vi "Copy .LLB to NI VeriStand dir.vi"(5 "Files Generated by Build":path[](array[path]), 6 "Top Level/Always Included VIs":path[](array[path]), 7 "Destination Path":path, 8 "error in (no error)":errorcluster, 9 "Target Name":string, 10 "Build Specification Name":string, 11 "Project Path":path) -> (0 "error out":errorcluster)   [LabVIEW 2024]
doc: "This VI is called after each run of a build specification. The VI will copy the generated LLB (Engine or System Explorer) into the VeriStand Custom Device folder (...\\Documents\\National Instruments\\NI VeriStand 2013...)."
uses:
  NationalInstruments.VeriStand
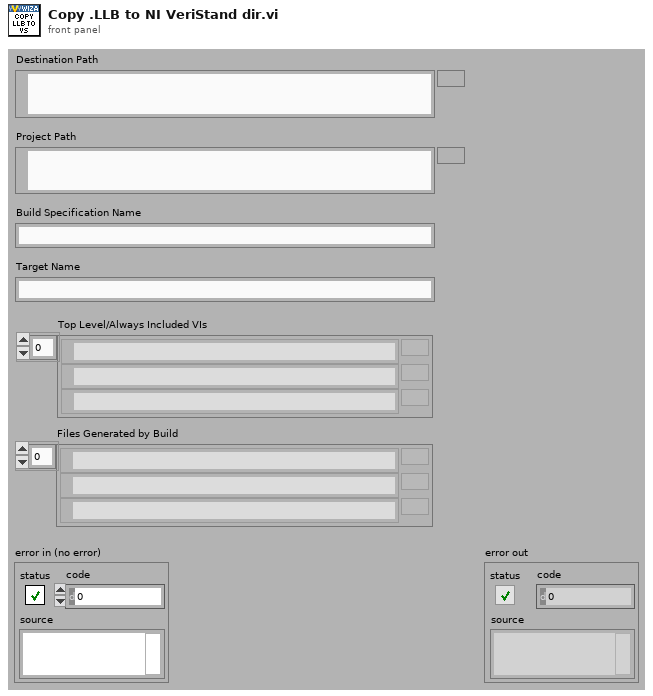
[diagram p1: front panel]
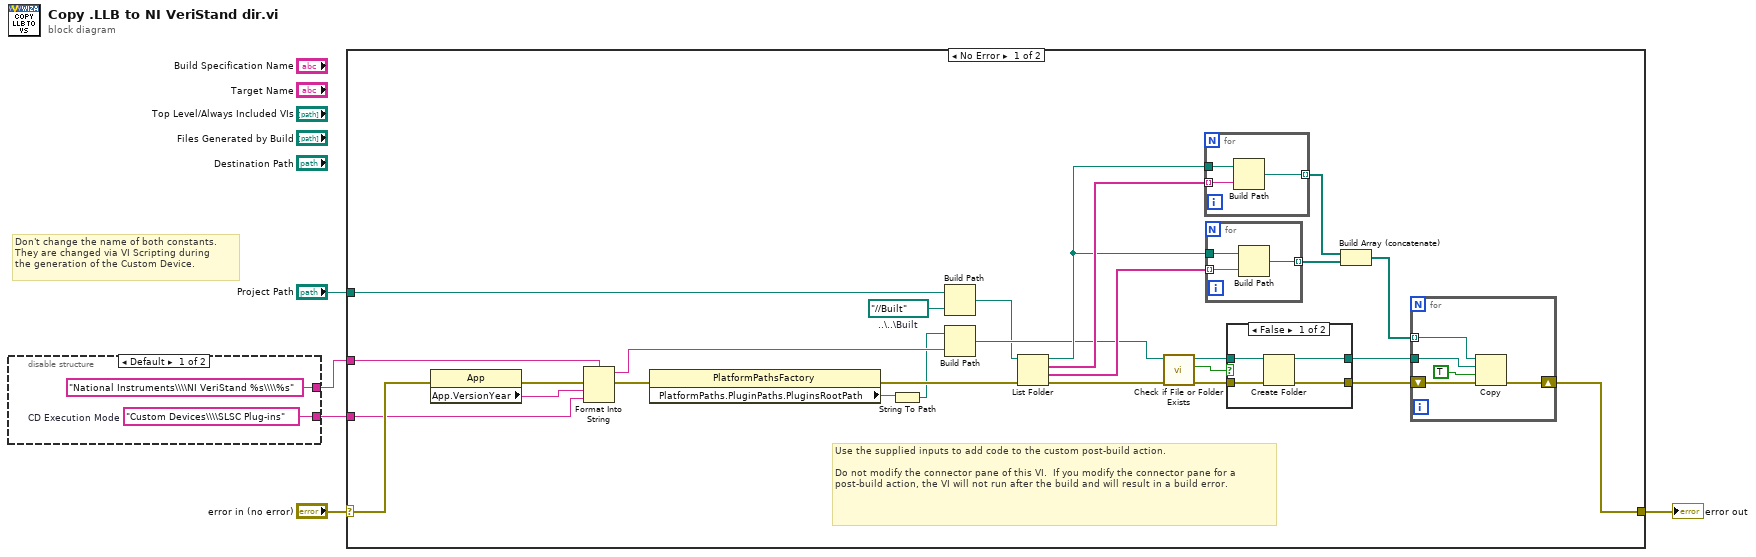
[diagram p0: block diagram]
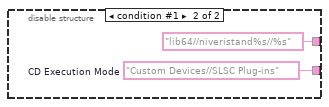
[diagram p4: hidden frame]
diagram:
  # "Don't change the name of both constants.\nThey are changed via VI Scripting during\nthe generation of the Custom Device."
  n1 = disable-structure shown="Default" {
    disable-tunnel: [w7 w9] -> w2
    disable-tunnel: ["National Instruments\\\\NI VeriStand %s\\\\%s" ("name or relative path") "lib64//niveristand%s//%s" ("name or relative path")] -> w1
    frame condition #0 (active) {
      w7 = "Custom Devices\\\\SLSC Plug-ins"  # CD Execution Mode
    }
    frame condition #1 {
      w9 = "Custom Devices//SLSC Plug-ins"  # CD Execution Mode
    }
  }
  n2 = case shown="No Error" "error in (no error)" {
    selector: "error in (no error)" -> [w22 w54]
    tunnel: [w24 w54] -> w3
    tunnel: "Project Path" -> [w21 _]
    tunnel: w2 -> [w16 _]
    tunnel: w1 -> [w14 _]
    frame No Error {
      w15 = path "../../Built"  # ..\..\Built
      # "Use the supplied inputs to add code to the custom post-build action.\n\nDo not modify the connector pane of this VI.  If you modify the connector pane for a post-build action, the VI will not run after the build and will result in a build error."
      n3 = property class="App"(error in=w22) -> (error out=w25:errorcluster, "App.VersionYear"=w17:string)  [unwired: 1 in, 1 out]
      n4 = Format Into String(format string=w14, error in=w25, w17, w16) -> (resulting string=w26:string, error out=w13:errorcluster)  [unwired: 1 in]
      n5 = property class="PlatformPathsFactory"(error in=w13) -> (error out=w12:errorcluster, "PlatformPaths.PluginPaths.PluginsRootPath"=w11:string)  [unwired: 1 in, 1 out]
      n6 = String To Path(string=w11) -> (path=w10:path)
      n7 = Build Path(base path=w21, name or relative path=w15) -> (appended path=w18:path)
      n8 = Build Path(base path=w10, name or relative path=w26) -> (appended path=w23:path)
      n9 = List Folder(path=w18, error in=w12) -> (path out=w29:path, filenames=w36:string[], folder names=w30:string[], error out=w27:errorcluster)  [unwired: 2 in]
      n10 = call <vilib>:"Check if File or Folder Exists.vi"("error in (no error)"=w27, "path"=w23) -> ("error out"=w31:errorcluster, "file or folder exists?"=w33:bool, "dup path"=w32:path)  [unwired: 7 in]
      n11 = for {
        tunnel: w36 -> [w52] mode=indexing
        tunnel: w29 -> [w53]
        tunnel: [w51] -> w35 mode=indexing
        n12 = Build Path(base path=w53, name or relative path=w52) -> (appended path=w51:path)
      }
      n13 = for {
        tunnel: w30 -> [w49] mode=indexing
        tunnel: w29 -> [w50]
        tunnel: [w48] -> w28 mode=indexing
        n14 = Build Path(base path=w50, name or relative path=w49) -> (appended path=w48:path)
      }
      n15 = case shown="False" w33 {
        tunnel: w32 -> [w40 w42]
        tunnel: w31 -> [w39 w41]
        tunnel: [w38 w42] -> w20
        tunnel: [w37 w41] -> w19
        frame False {
          n16 = Create Folder(path (use dialog)=w40, error in=w39) -> (created path=w38:path, error out=w37:errorcluster)  [unwired: 1 in, 1 out]
        }
        frame True {
        }
      }
      n17 = Build Array (concatenate)(w35, w28) -> (w34:path[])
      n18 = for {
        tunnel: w34 -> [w44] mode=indexing
        shift-right: [w45] -> w24
        shift-left: w19 -> [w46]
        tunnel: w20 -> [w43]
        n19 = Copy(8:w46, 9:TRUE ("overwrite (F)"), 10:w43, 11:w44) -> (0:w45:errorcluster)  [unwired: 1 in, 2 out]
      }
    }
    frame Error {
    }
  }
  "error out" <- w3
